vi "Create SE Zip EXE.vi"(8 "error in (no error)":errorcluster, 9 "Setup Dialog Text (\"\")":string, 10 "Source File/Directory":path, 11 "ZIP Archive Path (empty)":path) -> (0 "error out":errorcluster)   [LabVIEW 2011]
uses:
  OpenG/file/file.llb/Convert File Extension (Path)__ogtk.vi
panel:
  out "command":string
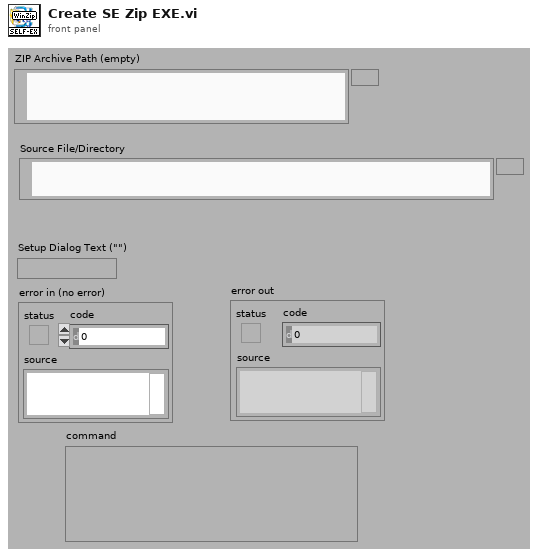
[diagram p1: front panel]
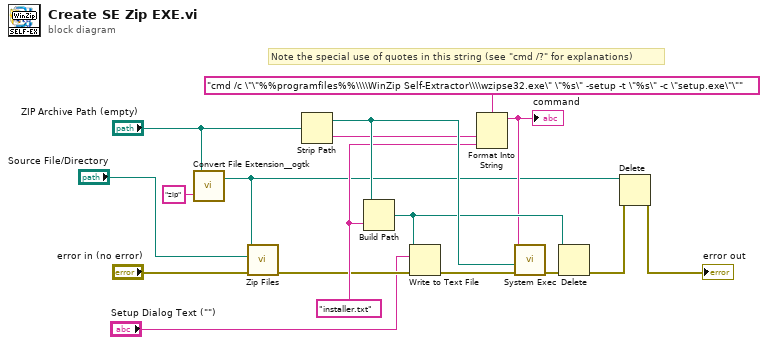
[diagram p0: block diagram]
diagram:
  w13 = "installer.txt" ("format string")
  # "Note the special use of quotes in this string (see \"cmd /?\" for explanations)"
  n1 = call-poly "Convert File Extension__ogtk.vi"("new ending (none)"="zip", "file name"="ZIP Archive Path (empty)") -> ("new filename"=w3:path)  [unwired: 1 out]
  n2 = call "Zip Files.vi"("error in (no error)"="error in (no error)", "Source File/Directory"="Source File/Directory", "Target Zip File"=w3) -> ("error out"=w8:errorcluster)  [unwired: 8 out]
  n3 = Strip Path(path="ZIP Archive Path (empty)") -> (stripped path=w14:path, name=w10:string)
  n4 = Build Path(base path=w14, name or relative path=w13) -> (appended path=w12:path)
  n5 = Write to Text File(file (use dialog)=w12, text="Setup Dialog Text (\"\")", error in=w8) -> (error out=w16:errorcluster)  [unwired: 3 out]
  n6 = Format Into String(format string="cmd /c \"\"%%programfiles%%\\\\WinZip Self-Extractor\\\\wzipse32.exe\" \"%s\" -setup -t \"%s\" -c \"setup.exe\"\"", w10, w13) -> (resulting string=w11:string)  [unwired: 2 in, 1 out]
  "command" <- w11
  n7 = call <vilib>:"System Exec.vi"("error in (no error)"=w16, "working directory"=w14, "command line"=w11) -> ("error out"=w15:errorcluster)  [unwired: 3 in, 5 out]
  n8 = Delete(path (use dialog)=w12, error in=w15) -> (error out=w2:errorcluster)  [unwired: 5 out]
  n9 = Delete(path (use dialog)=w3, error in=w2) -> (error out=→"error out":errorcluster)  [unwired: 5 out]
